vi "FTW-Test-JSON-Equality.vi"() -> ()   [LabVIEW 2015]
uses:
  source/container/FTW-Container.lvclass
panel:
  out "Equal":bool
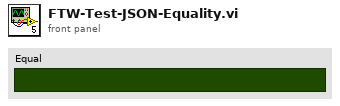
[diagram p1: front panel]
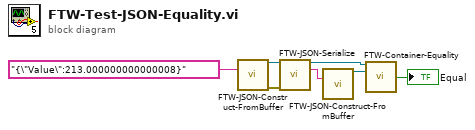
[diagram p0: block diagram]
diagram:
  n1 = call "FTW-JSON-Construct-FromBuffer.vi"("JSON String (UTF-8)"="{\"Value\":213.000000000000008}") -> ("JSON"=w6:refnum<class "FTW-Container.lvclass">, "error out"=w5:errorcluster)  [unwired: 13 in]
  n2 = call "FTW-JSON-Serialize.vi"("JSON"=w6, "error in"=w5) -> ("JSON out"=w3:refnum<class "FTW-Container.lvclass">, "JSON String (UTF-8)"=w4:string)  [unwired: 11 in, 1 out]
  n3 = call "FTW-JSON-Construct-FromBuffer.vi"("JSON String (UTF-8)"=w4) -> ("JSON"=w2:refnum<class "FTW-Container.lvclass">)  [unwired: 13 in, 1 out]
  n4 = call "FTW-Container-Equality.vi"("FTW-Container In"=w3, "Other Container"=w2) -> ("Equal"=→"Equal":bool)  [unwired: 11 in, 2 out]
